vi "App - analyze RUS V6.vi"() -> ()   [LabVIEW 2021] (continued)
format"=enum."binary", "power(V)"=2.1, "Magn Field(T) "=0.0}, {"temperature"=67.561, "temperature str"="67.56100", "file path"=path "D:/Data/Ultrasound/LSCO/LSCO22__130814c/5_Cooling_2nd_try/September_2014/091714/67.56100K_500_2500_2.10000V_0.00000T_Sep17-2014__05-35-15_001_091714.bin", "last mod"=timestamp(3493791315 s since 1904-01-01), "file name str"="D:\\Data\\Ultrasound\\LSCO\\LSCO22__130814c\\5_Cooling_2nd_try\\September_2014\\091714\\67.56100K_500_2500_2.10000V_0.00000T_Sep17-2014__05-35-15_001_091714.bin", "mod time(min)"=58229855.25, "file format"=enum."binary", "power(V)"=2.1, "Magn Field(T) "=0.0}, {"temperature"=67.503, "temperature str"="67.50300", "file path"=path "D:/Data/Ultrasound/LSCO/LSCO22__130814c/5_Cooling_2nd_try/September_2014/091714/67.50300K_500_2500_2.10000V_0.00000T_Sep17-2014__05-36-34_001_091714.bin", "last mod"=timestamp(3493791394 s since 1904-01-01), "file name str"="D:\\Data\\Ultrasound\\LSCO\\LSCO22__130814c\\5_Cooling_2nd_try\\September_2014\\091714\\67.50300K_500_2500_2.10000V_0.00000T_Sep17-2014__05-36-34_001_091714.bin", "mod time(min)"=58229856.56666667, "file format"=enum."binary", "power(V)"=2.1, "Magn Field(T) "=0.0}, {"temperature"=67.441, "temperature str"="67.44100", "file path"=path "D:/Data/Ultrasound/LSCO/LSCO22__130814c/5_Cooling_2nd_try/September_2014/091714/67.44100K_500_2500_2.10000V_0.00000T_Sep17-2014__05-37-53_001_091714.bin", "last mod"=timestamp(3493791473 s since 1904-01-01), "file name str"="D:\\Data\\Ultrasound\\LSCO\\LSCO22__130814c\\5_Cooling_2nd_try\\September_2014\\091714\\67.44100K_500_2500_2.10000V_0.00000T_Sep17-2014__05-37-53_001_091714.bin", "mod time(min)"=58229857.88333333, "file format"=enum."binary", "power(V)"=2.1, "Magn Field(T) "=0.0}, {"temperature"=67.379, "temperature str"="67.37900", "file path"=path "D:/Data/Ultrasound/LSCO/LSCO22__130814c/5_Cooling_2nd_try/September_2014/091714/67.37900K_500_2500_2.10000V_0.00000T_Sep17-2014__05-39-13_001_091714.bin", "last mod"=timestamp(3493791553 s since 1904-01-01), "file name str"="D:\\Data\\Ultrasound\\LSCO\\LSCO22__130814c\\5_Cooling_2nd_try\\September_2014\\091714\\67.37900K_500_2500_2.10000V_0.00000T_Sep17-2014__05-39-13_001_091714.bin", "mod time(min)"=58229859.21666667, "file format"=enum."binary", "power(V)"=2.1, "Magn Field(T) "=0.0}, {"temperature"=67.322, "temperature str"="67.32200", "file path"=path "D:/Data/Ultrasound/LSCO/LSCO22__130814c/5_Cooling_2nd_try/September_2014/091714/67.32200K_500_2500_2.10000V_0.00000T_Sep17-2014__05-40-32_001_091714.bin", "last mod"=timestamp(3493791632 s since 1904-01-01), "file name str"="D:\\Data\\Ultrasound\\LSCO\\LSCO22__130814c\\5_Cooling_2nd_try\\September_2014\\091714\\67.32200K_500_2500_2.10000V_0.00000T_Sep17-2014__05-40-32_001_091714.bin", "mod time(min)"=58229860.53333333, "file format"=enum."binary", "power(V)"=2.1, "Magn Field(T) "=0.0}, {"temperature"=67.261, "temperature str"="67.26100", "file path"=path "D:/Data/Ultrasound/LSCO/LSCO22__130814c/5_Cooling_2nd_try/September_2014/091714/67.26100K_500_2500_2.10000V_0.00000T_Sep17-2014__05-41-51_001_091714.bin", "last mod"=timestamp(3493791711 s since 1904-01-01), "file name str"="D:\\Data\\Ultrasound\\LSCO\\LSCO22__130814c\\5_Cooling_2nd_try\\September_2014\\091714\\67.26100K_500_2500_2.10000V_0.00000T_Sep17-2014__05-41-51_001_091714.bin", "mod time(min)"=58229861.85, "file format"=enum."binary", "power(V)"=2.1, "Magn Field(T) "=0.0}, {"temperature"=67.202, "temperature str"="67.20200", "file path"=path "D:/Data/Ultrasound/LSCO/LSCO22__130814c/5_Cooling_2nd_try/September_2014/091714/67.20200K_500_2500_2.10000V_0.00000T_Sep17-2014__05-43-11_001_091714.bin", "last mod"=timestamp(3493791791 s since 1904-01-01), "file name str"="D:\\Data\\Ultrasound\\LSCO\\LSCO22__130814c\\5_Cooling_2nd_try\\September_2014\\091714\\67.20200K_500_2500_2.10000V_0.00000T_Sep17-2014__05-43-11_001_091714.bin", "mod time(min)"=58229863.18333333, "file format"=enum."binary", "power(V)"=2.1, "Magn Field(T) "=0.0}, {"temperature"=67.139, "temperature str"="67.13900", "file path"=path "D:/Data/Ultrasound/LSCO/LSCO22__130814c/5_Cooling_2nd_try/September_2014/091714/67.13900K_500_2500_2.10000V_0.00000T_Sep17-2014__05-44-30_001_091714.bin", "last mod"=timestamp(3493791870 s since 1904-01-01), "file name str"="D:\\Data\\Ultrasound\\LSCO\\LSCO22__130814c\\5_Cooling_2nd_try\\September_2014\\091714\\67.13900K_500_2500_2.10000V_0.00000T_Sep17-2014__05-44-30_001_091714.bin", "mod time(min)"=58229864.5, "file format"=enum."binary", "power(V)"=2.1, "Magn Field(T) "=0.0}, {"temperature"=67.079, "temperature str"="67.07900", "file path"=path "D:/Data/Ultrasound/LSCO/LSCO22__130814c/5_Cooling_2nd_try/September_2014/091714/67.07900K_500_2500_2.10000V_0.00000T_Sep17-2014__05-45-49_001_091714.bin", "last mod"=timestamp(3493791949 s since 1904-01-01), "file name str"="D:\\Data\\Ultrasound\\LSCO\\LSCO22__130814c\\5_Cooling_2nd_try\\September_2014\\091714\\67.07900K_500_2500_2.10000V_0.00000T_Sep17-2014__05-45-49_001_091714.bin", "mod time(min)"=58229865.81666667, "file format"=enum."binary", "power(V)"=2.1, "Magn Field(T) "=0.0}, {"temperature"=67.02, "temperature str"="67.02000", "file path"=path "D:/Data/Ultrasound/LSCO/LSCO22__130814c/5_Cooling_2nd_try/September_2014/091714/67.02000K_500_2500_2.10000V_0.00000T_Sep17-2014__05-47-09_001_091714.bin", "last mod"=timestamp(3493792029 s since 1904-01-01), "file name str"="D:\\Data\\Ultrasound\\LSCO\\LSCO22__130814c\\5_Cooling_2nd_try\\September_2014\\091714\\67.02000K_500_2500_2.10000V_0.00000T_Sep17-2014__05-47-09_001_091714.bin", "mod time(min)"=58229867.15, "file format"=enum."binary", "power(V)"=2.1, "Magn Field(T) "=0.0}, {"temperature"=66.959, "temperature str"="66.95900", "file path"=path "D:/Data/Ultrasound/LSCO/LSCO22__130814c/5_Cooling_2nd_try/September_2014/091714/66.95900K_500_2500_2.10000V_0.00000T_Sep17-2014__05-48-28_001_091714.bin", "last mod"=timestamp(3493792108 s since 1904-01-01), "file name str"="D:\\Data\\Ultrasound\\LSCO\\LSCO22__130814c\\5_Cooling_2nd_try\\September_2014\\091714\\66.95900K_500_2500_2.10000V_0.00000T_Sep17-2014__05-48-28_001_091714.bin", "mod time(min)"=58229868.46666667, "file format"=enum."binary", "power(V)"=2.1, "Magn Field(T) "=0.0}, {"temperature"=66.901, "temperature str"="66.90100", "file path"=path "D:/Data/Ultrasound/LSCO/LSCO22__130814c/5_Cooling_2nd_try/September_2014/091714/66.90100K_500_2500_2.10000V_0.00000T_Sep17-2014__05-49-47_001_091714.bin", "last mod"=timestamp(3493792187 s since 1904-01-01), "file name str"="D:\\Data\\Ultrasound\\LSCO\\LSCO22__130814c\\5_Cooling_2nd_try\\September_2014\\091714\\66.90100K_500_2500_2.10000V_0.00000T_Sep17-2014__05-49-47_001_091714.bin", "mod time(min)"=58229869.78333333, "file format"=enum."binary", "power(V)"=2.1, "Magn Field(T) "=0.0}, {"temperature"=66.841, "temperature str"="66.84100", "file path"=path "D:/Data/Ultrasound/LSCO/LSCO22__130814c/5_Cooling_2nd_try/September_2014/091714/66.84100K_500_2500_2.10000V_0.00000T_Sep17-2014__05-51-07_001_091714.bin", "last mod"=timestamp(3493792267 s since 1904-01-01), "file name str"="D:\\Data\\Ultrasound\\LSCO\\LSCO22__130814c\\5_Cooling_2nd_try\\September_2014\\091714\\66.84100K_500_2500_2.10000V_0.00000T_Sep17-2014__05-51-07_001_091714.bin", "mod time(min)"=58229871.11666667, "file format"=enum."binary", "power(V)"=2.1, "Magn Field(T) "=0.0}, {"temperature"=66.779, "temperature str"="66.77900", "file path"=path "D:/Data/Ultrasound/LSCO/LSCO22__130814c/5_Cooling_2nd_try/September_2014/091714/66.77900K_500_2500_2.10000V_0.00000T_Sep17-2014__05-52-26_001_091714.bin", "last mod"=timestamp(3493792346 s since 1904-01-01), "file name str"="D:\\Data\\Ultrasound\\LSCO\\LSCO22__130814c\\5_Cooling_2nd_try\\September_2014\\091714\\66.77900K_500_2500_2.10000V_0.00000T_Sep17-2014__05-52-26_001_091714.bin", "mod time(min)"=58229872.43333333, "file format"=enum."binary", "power(V)"=2.1, "Magn Field(T) "=0.0}, {"temperature"=66.721, "temperature str"="66.72100", "file path"=path "D:/Data/Ultrasound/LSCO/LSCO22__130814c/5_Cooling_2nd_try/September_2014/091714/66.72100K_500_2500_2.10000V_0.00000T_Sep17-2014__05-53-45_001_091714.bin", "last mod"=timestamp(3493792425 s since 1904-01-01), "file name str"="D:\\Data\\Ultrasound\\LSCO\\LSCO22__130814c\\5_Cooling_2nd_try\\September_2014\\091714\\66.72100K_500_2500_2.10000V_0.00000T_Sep17-2014__05-53-45_001_091714.bin", "mod time(min)"=58229873.75, "file format"=enum."binary", "power(V)"=2.1, "Magn Field(T) "=0.0}, {"temperature"=66.66, "temperature str"="66.66000", "file path"=path "D:/Data/Ultrasound/LSCO/LSCO22__130814c/5_Cooling_2nd_try/September_2014/091714/66.66000K_500_2500_2.10000V_0.00000T_Sep17-2014__05-55-05_001_091714.bin", "last mod"=timestamp(3493792505 s since 1904-01-01), "file name str"="D:\\Data\\Ultrasound\\LSCO\\LSCO22__130814c\\5_Cooling_2nd_try\\September_2014\\091714\\66.66000K_500_2500_2.10000V_0.00000T_Sep17-2014__05-55-05_001_091714.bin", "mod time(min)"=58229875.083333336, "file format"=enum."binary", "power(V)"=2.1, "Magn Field(T) "=0.0}, {"temperature"=66.601, "temperature str"="66.60100", "file path"=path "D:/Data/Ultrasound/LSCO/LSCO22__130814c/5_Cooling_2nd_try/September_2014/091714/66.60100K_500_2500_2.10000V_0.00000T_Sep17-2014__05-56-24_001_091714.bin", "last mod"=timestamp(3493792584 s since 1904-01-01), "file name str"="D:\\Data\\Ultrasound\\LSCO\\LSCO22__130814c\\5_Cooling_2nd_try\\September_2014\\091714\\66.60100K_500_2500_2.10000V_0.00000T_Sep17-2014__05-56-24_001_091714.bin", "mod time(min)"=58229876.4, "file format"=enum."binary", "power(V)"=2.1, "Magn Field(T) "=0.0}, {"temperature"=66.541, "temperature str"="66.54100", "file path"=path "D:/Data/Ultrasound/LSCO/LSCO22__130814c/5_Cooling_2nd_try/September_2014/091714/66.54100K_500_2500_2.10000V_0.00000T_Sep17-2014__05-57-44_001_091714.bin", "last mod"=timestamp(3493792664 s since 1904-01-01), "file name str"="D:\\Data\\Ultrasound\\LSCO\\LSCO22__130814c\\5_Cooling_2nd_try\\September_2014\\091714\\66.54100K_500_2500_2.10000V_0.00000T_Sep17-2014__05-57-44_001_091714.bin", "mod time(min)"=58229877.733333334, "file format"=enum."binary", "power(V)"=2.1, "Magn Field(T) "=0.0}, {"temperature"=66.48, "temperature str"="66.48000", "file path"=path "D:/Data/Ultrasound/LSCO/LSCO22__130814c/5_Cooling_2nd_try/September_2014/091714/66.48000K_500_2500_2.10000V_0.00000T_Sep17-2014__05-59-03_001_091714.bin", "last mod"=timestamp(3493792743 s since 1904-01-01), "file name str"="D:\\Data\\Ultrasound\\LSCO\\LSCO22__130814c\\5_Cooling_2nd_try\\September_2014\\091714\\66.48000K_500_2500_2.10000V_0.00000T_Sep17-2014__05-59-03_001_091714.bin", "mod time(min)"=58229879.05, "file format"=enum."binary", "power(V)"=2.1, "Magn Field(T) "=0.0}, {"temperature"=66.422, "temperature str"="66.42200", "file path"=path "D:/Data/Ultrasound/LSCO/LSCO22__130814c/5_Cooling_2nd_try/September_2014/091714/66.42200K_500_2500_2.10000V_0.00000T_Sep17-2014__06-00-22_001_091714.bin", "last mod"=timestamp(3493792822 s since 1904-01-01), "file name str"="D:\\Data\\Ultrasound\\LSCO\\LSCO22__130814c\\5_Cooling_2nd_try\\September_2014\\091714\\66.42200K_500_2500_2.10000V_0.00000T_Sep17-2014__06-00-22_001_091714.bin", "mod time(min)"=58229880.36666667, "file format"=enum."binary", "power(V)"=2.1, "Magn Field(T) "=0.0}, {"temperature"=66.363, "temperature str"="66.36300", "file path"=path "D:/Data/Ultrasound/LSCO/LSCO22__130814c/5_Cooling_2nd_try/September_2014/091714/66.36300K_500_2500_2.10000V_0.00000T_Sep17-2014__06-01-42_001_091714.bin", "last mod"=timestamp(3493792902 s since 1904-01-01), "file name str"="D:\\Data\\Ultrasound\\LSCO\\LSCO22__130814c\\5_Cooling_2nd_try\\September_2014\\091714\\66.36300K_500_2500_2.10000V_0.00000T_Sep17-2014__06-01-42_001_091714.bin", "mod time(min)"=58229881.7, "file format"=enum."binary", "power(V)"=2.1, "Magn Field(T) "=0.0}, {"temperature"=66.302, "temperature str"="66.30200", "file path"=path "D:/Data/Ultrasound/LSCO/LSCO22__130814c/5_Cooling_2nd_try/September_2014/091714/66.30200K_500_2500_2.10000V_0.00000T_Sep17-2014__06-03-01_001_091714.bin", "last mod"=timestamp(3493792981 s since 1904-01-01), "file name str"="D:\\Data\\Ultrasound\\LSCO\\LSCO22__130814c\\5_Cooling_2nd_try\\September_2014\\091714\\66.30200K_500_2500_2.10000V_0.00000T_Sep17-2014__06-03-01_001_091714.bin", "mod time(min)"=58229883.016666666, "file format"=enum."binary", "power(V)"=2.1, "Magn Field(T) "=0.0}, {"temperature"=66.244, "temperature str"="66.24400", "file path"=path "D:/Data/Ultrasound/LSCO/LSCO22__130814c/5_Cooling_2nd_try/September_2014/091714/66.24400K_500_2500_2.10000V_0.00000T_Sep17-2014__06-04-20_001_091714.bin", "last mod"=timestamp(3493793060 s since 1904-01-01), "file name str"="D:\\Data\\Ultrasound\\LSCO\\LSCO22__130814c\\5_Cooling_2nd_try\\September_2014\\091714\\66.24400K_500_2500_2.10000V_0.00000T_Sep17-2014__06-04-20_001_091714.bin", "mod time(min)"=58229884.333333336, "file format"=enum."binary", "power(V)"=2.1, "Magn Field(T) "=0.0}, {"temperature"=66.182, "temperature str"="66.18200", "file path"=path "D:/Data/Ultrasound/LSCO/LSCO22__130814c/5_Cooling_2nd_try/September_2014/091714/66.18200K_500_2500_2.10000V_0.00000T_Sep17-2014__06-05-40_001_091714.bin", "last mod"=timestamp(3493793140 s since 1904-01-01), "file name str"="D:\\Data\\Ultrasound\\LSCO\\LSCO22__130814c\\5_Cooling_2nd_try\\September_2014\\091714\\66.18200K_500_2500_2.10000V_0.00000T_Sep17-2014__06-05-40_001_091714.bin", "mod time(min)"=58229885.666666664, "file format"=enum."binary", "power(V)"=2.1, "Magn Field(T) "=0.0}, {"temperature"=66.124, "temperature str"="66.12400", "file path"=path "D:/Data/Ultrasound/LSCO/LSCO22__130814c/5_Cooling_2nd_try/September_2014/091714/66.12400K_500_2500_2.10000V_0.00000T_Sep17-2014__06-06-59_001_091714.bin", "last mod"=timestamp(3493793219 s since 1904-01-01), "file name str"="D:\\Data\\Ultrasound\\LSCO\\LSCO22__130814c\\5_Cooling_2nd_try\\September_2014\\091714\\66.12400K_500_2500_2.10000V_0.00000T_Sep17-2014__06-06-59_001_091714.bin", "mod time(min)"=58229886.983333334, "file format"=enum."binary", "power(V)"=2.1, "Magn Field(T) "=0.0}, {"temperature"=66.063, "temperature str"="66.06300", "file path"=path "D:/Data/Ultrasound/LSCO/LSCO22__130814c/5_Cooling_2nd_try/September_2014/091714/66.06300K_500_2500_2.10000V_0.00000T_Sep17-2014__06-08-19_001_091714.bin", "last mod"=timestamp(3493793299 s since 1904-01-01), "file name str"="D:\\Data\\Ultrasound\\LSCO\\LSCO22__130814c\\5_Cooling_2nd_try\\September_2014\\091714\\66.06300K_500_2500_2.10000V_0.00000T_Sep17-2014__06-08-19_001_091714.bin", "mod time(min)"=58229888.31666667, "file format"=enum."binary", "power(V)"=2.1, "Magn Field(T) "=0.0}, {"temperature"=66.006, "temperature str"="66.00600", "file path"=path "D:/Data/Ultrasound/LSCO/LSCO22__130814c/5_Cooling_2nd_try/September_2014/091714/66.00600K_500_2500_2.10000V_0.00000T_Sep17-2014__06-09-38_001_091714.bin", "last mod"=timestamp(3493793378 s since 1904-01-01), "file name str"="D:\\Data\\Ultrasound\\LSCO\\LSCO22__130814c\\5_Cooling_2nd_try\\September_2014\\091714\\66.00600K_500_2500_2.10000V_0.00000T_Sep17-2014__06-09-38_001_091714.bin", "mod time(min)"=58229889.63333333, "file format"=enum."binary", "power(V)"=2.1, "Magn Field(T) "=0.0}, {"temperature"=65.947, "temperature str"="65.94700", "file path"=path "D:/Data/Ultrasound/LSCO/LSCO22__130814c/5_Cooling_2nd_try/September_2014/091714/65.94700K_500_2500_2.10000V_0.00000T_Sep17-2014__06-10-57_001_091714.bin", "last mod"=timestamp(3493793457 s since 1904-01-01), "file name str"="D:\\Data\\Ultrasound\\LSCO\\LSCO22__130814c\\5_Cooling_2nd_try\\September_2014\\091714\\65.94700K_500_2500_2.10000V_0.00000T_Sep17-2014__06-10-57_001_091714.bin", "mod time(min)"=58229890.95, "file format"=enum."binary", "power(V)"=2.1, "Magn Field(T) "=0.0}, {"temperature"=65.884, "temperature str"="65.88400", "file path"=path "D:/Data/Ultrasound/LSCO/LSCO22__130814c/5_Cooling_2nd_try/September_2014/091714/65.88400K_500_2500_2.10000V_0.00000T_Sep17-2014__06-12-17_001_091714.bin", "last mod"=timestamp(3493793537 s since 1904-01-01), "file name str"="D:\\Data\\Ultrasound\\LSCO\\LSCO22__130814c\\5_Cooling_2nd_try\\September_2014\\091714\\65.88400K_500_2500_2.10000V_0.00000T_Sep17-2014__06-12-17_001_091714.bin", "mod time(min)"=58229892.28333333, "file format"=enum."binary", "power(V)"=2.1, "Magn Field(T) "=0.0}, {"temperature"=65.828, "temperature str"="65.82800", "file path"=path "D:/Data/Ultrasound/LSCO/LSCO22__130814c/5_Cooling_2nd_try/September_2014/091714/65.82800K_500_2500_2.10000V_0.00000T_Sep17-2014__06-13-36_001_091714.bin", "last mod"=timestamp(3493793616 s since 1904-01-01), "file name str"="D:\\Data\\Ultrasound\\LSCO\\LSCO22__130814c\\5_Cooling_2nd_try\\September_2014\\091714\\65.82800K_500_2500_2.10000V_0.00000T_Sep17-2014__06-13-36_001_091714.bin", "mod time(min)"=58229893.6, "file format"=enum."binary", "power(V)"=2.1, "Magn Field(T) "=0.0}, {"temperature"=65.767, "temperature str"="65.76700", "file path"=path "D:/Data/Ultrasound/LSCO/LSCO22__130814c/5_Cooling_2nd_try/September_2014/091714/65.76700K_500_2500_2.10000V_0.00000T_Sep17-2014__06-14-56_001_091714.bin", "last mod"=timestamp(3493793696 s since 1904-01-01), "file name str"="D:\\Data\\Ultrasound\\LSCO\\LSCO22__130814c\\5_Cooling_2nd_try\\September_2014\\091714\\65.76700K_500_2500_2.10000V_0.00000T_Sep17-2014__06-14-56_001_091714.bin", "mod time(min)"=58229894.93333333, "file format"=enum."binary", "power(V)"=2.1, "Magn Field(T) "=0.0}, {"temperature"=65.71, "temperature str"="65.71000", "file path"=path "D:/Data/Ultrasound/LSCO/LSCO22__130814c/5_Cooling_2nd_try/September_2014/091714/65.71000K_500_2500_2.10000V_0.00000T_Sep17-2014__06-16-15_001_091714.bin", "last mod"=timestamp(3493793775 s since 1904-01-01), "file name str"="D:\\Data\\Ultrasound\\LSCO\\LSCO22__130814c\\5_Cooling_2nd_try\\September_2014\\091714\\65.71000K_500_2500_2.10000V_0.00000T_Sep17-2014__06-16-15_001_091714.bin", "mod time(min)"=58229896.25, "file format"=enum."binary", "power(V)"=2.1, "Magn Field(T) "=0.0}, {"temperature"=65.648, "temperature str"="65.64800", "file path"=path "D:/Data/Ultrasound/LSCO/LSCO22__130814c/5_Cooling_2nd_try/September_2014/091714/65.64800K_500_2500_2.10000V_0.00000T_Sep17-2014__06-17-34_001_091714.bin", "last mod"=timestamp(3493793854 s since 1904-01-01), "file name str"="D:\\Data\\Ultrasound\\LSCO\\LSCO22__130814c\\5_Cooling_2nd_try\\September_2014\\091714\\65.64800K_500_2500_2.10000V_0.00000T_Sep17-2014__06-17-34_001_091714.bin", "mod time(min)"=58229897.56666667, "file format"=enum."binary", "power(V)"=2.1, "Magn Field(T) "=0.0}, {"temperature"=65.588, "temperature str"="65.58800", "file path"=path "D:/Data/Ultrasound/LSCO/LSCO22__130814c/5_Cooling_2nd_try/September_2014/091714/65.58800K_500_2500_2.10000V_0.00000T_Sep17-2014__06-18-54_001_091714.bin", "last mod"=timestamp(3493793934 s since 1904-01-01), "file name str"="D:\\Data\\Ultrasound\\LSCO\\LSCO22__130814c\\5_Cooling_2nd_try\\September_2014\\091714\\65.58800K_500_2500_2.10000V_0.00000T_Sep17-2014__06-18-54_001_091714.bin", "mod time(min)"=58229898.9, "file format"=enum."binary", "power(V)"=2.1, "Magn Field(T) "=0.0}, {"temperature"=65.531, "temperature str"="65.53100", "file path"=path "D:/Data/Ultrasound/LSCO/LSCO22__130814c/5_Cooling_2nd_try/September_2014/091714/65.53100K_500_2500_2.10000V_0.00000T_Sep17-2014__06-20-13_001_091714.bin", "last mod"=timestamp(3493794013 s since 1904-01-01), "file name str"="D:\\Data\\Ultrasound\\LSCO\\LSCO22__130814c\\5_Cooling_2nd_try\\September_2014\\091714\\65.53100K_500_2500_2.10000V_0.00000T_Sep17-2014__06-20-13_001_091714.bin", "mod time(min)"=58229900.21666667, "file format"=enum."binary", "power(V)"=2.1, "Magn Field(T) "=0.0}, {"temperature"=65.472, "temperature str"="65.47200", "file path"=path "D:/Data/Ultrasound/LSCO/LSCO22__130814c/5_Cooling_2nd_try/September_2014/091714/65.47200K_500_2500_2.10000V_0.00000T_Sep17-2014__06-21-32_001_091714.bin", "last mod"=timestamp(3493794092 s since 1904-01-01), "file name str"="D:\\Data\\Ultrasound\\LSCO\\LSCO22__130814c\\5_Cooling_2nd_try\\September_2014\\091714\\65.47200K_500_2500_2.10000V_0.00000T_Sep17-2014__06-21-32_001_091714.bin", "mod time(min)"=58229901.53333333, "file format"=enum."binary", "power(V)"=2.1, "Magn Field(T) "=0.0}, {"temperature"=65.412, "temperature str"="65.41200", "file path"=path "D:/Data/Ultrasound/LSCO/LSCO22__130814c/5_Cooling_2nd_try/September_2014/091714/65.41200K_500_2500_2.10000V_0.00000T_Sep17-2014__06-22-52_001_091714.bin", "last mod"=timestamp(3493794172 s since 1904-01-01), "file name str"="D:\\Data\\Ultrasound\\LSCO\\LSCO22__130814c\\5_Cooling_2nd_try\\September_2014\\091714\\65.41200K_500_2500_2.10000V_0.00000T_Sep17-2014__06-22-52_001_091714.bin", "mod time(min)"=58229902.86666667, "file format"=enum."binary", "power(V)"=2.1, "Magn Field(T) "=0.0}, {"temperature"=65.354, "temperature str"="65.35400", "file path"=path "D:/Data/Ultrasound/LSCO/LSCO22__130814c/5_Cooling_2nd_try/September_2014/091714/65.35400K_500_2500_2.10000V_0.00000T_Sep17-2014__06-24-11_001_091714.bin", "last mod"=timestamp(3493794251 s since 1904-01-01), "file name str"="D:\\Data\\Ultrasound\\LSCO\\LSCO22__130814c\\5_Cooling_2nd_try\\September_2014\\091714\\65.35400K_500_2500_2.10000V_0.00000T_Sep17-2014__06-24-11_001_091714.bin", "mod time(min)"=58229904.18333333, "file format"=enum."binary", "power(V)"=2.1, "Magn Field(T) "=0.0}, {"temperature"=65.294, "temperature str"="65.29400", "file path"=path "D:/Data/Ultrasound/LSCO/LSCO22__130814c/5_Cooling_2nd_try/September_2014/091714/65.29400K_500_2500_2.10000V_0.00000T_Sep17-2014__06-25-31_001_091714.bin", "last mod"=timestamp(3493794331 s since 1904-01-01), "file name str"="D:\\Data\\Ultrasound\\LSCO\\LSCO22__130814c\\5_Cooling_2nd_try\\September_2014\\091714\\65.29400K_500_2500_2.10000V_0.00000T_Sep17-2014__06-25-31_001_091714.bin", "mod time(min)"=58229905.516666666, "file format"=enum."binary", "power(V)"=2.1, "Magn Field(T) "=0.0}, {"temperature"=65.236, "temperature str"="65.23600", "file path"=path "D:/Data/Ultrasound/LSCO/LSCO22__130814c/5_Cooling_2nd_try/September_2014/091714/65.23600K_500_2500_2.10000V_0.00000T_Sep17-2014__06-26-50_001_091714.bin", "last mod"=timestamp(3493794410 s since 1904-01-01), "file name str"="D:\\Data\\Ultrasound\\LSCO\\LSCO22__130814c\\5_Cooling_2nd_try\\September_2014\\091714\\65.23600K_500_2500_2.10000V_0.00000T_Sep17-2014__06-26-50_001_091714.bin", "mod time(min)"=58229906.833333336, "file format"=enum."binary", "power(V)"=2.1, "Magn Field(T) "=0.0}, {"temperature"=65.176, "temperature str"="65.17600", "file path"=path "D:/Data/Ultrasound/LSCO/LSCO22__130814c/5_Cooling_2nd_try/September_2014/091714/65.17600K_500_2500_2.10000V_0.00000T_Sep17-2014__06-28-09_001_091714.bin", "last mod"=timestamp(3493794489 s since 1904-01-01), "file name str"="D:\\Data\\Ultrasound\\LSCO\\LSCO22__130814c\\5_Cooling_2nd_try\\September_2014\\091714\\65.17600K_500_2500_2.10000V_0.00000T_Sep17-2014__06-28-09_001_091714.bin", "mod time(min)"=58229908.15, "file format"=enum."binary", "power(V)"=2.1, "Magn Field(T) "=0.0}, {"temperature"=65.115, "temperature str"="65.11500", "file path"=path "D:/Data/Ultrasound/LSCO/LSCO22__130814c/5_Cooling_2nd_try/September_2014/091714/65.11500K_500_2500_2.10000V_0.00000T_Sep17-2014__06-29-29_001_091714.bin", "last mod"=timestamp(3493794569 s since 1904-01-01), "file name str"="D:\\Data\\Ultrasound\\LSCO\\LSCO22__130814c\\5_Cooling_2nd_try\\September_2014\\091714\\65.11500K_500_2500_2.10000V_0.00000T_Sep17-2014__06-29-29_001_091714.bin", "mod time(min)"=58229909.483333334, "file format"=enum."binary", "power(V)"=2.1, "Magn Field(T) "=0.0}, {"temperature"=65.059, "temperature str"="65.05900", "file path"=path "D:/Data/Ultrasound/LSCO/LSCO22__130814c/5_Cooling_2nd_try/September_2014/091714/65.05900K_500_2500_2.10000V_0.00000T_Sep17-2014__06-30-48_001_091714.bin", "last mod"=timestamp(3493794648 s since 1904-01-01), "file name str"="D:\\Data\\Ultrasound\\LSCO\\LSCO22__130814c\\5_Cooling_2nd_try\\September_2014\\091714\\65.05900K_500_2500_2.10000V_0.00000T_Sep17-2014__06-30-48_001_091714.bin", "mod time(min)"=58229910.8, "file format"=enum."binary", "power(V)"=2.1, "Magn Field(T) "=0.0}, {"temperature"=64.997, "temperature str"="64.99700", "file path"=path "D:/Data/Ultrasound/LSCO/LSCO22__130814c/5_Cooling_2nd_try/September_2014/091714/64.99700K_500_2500_2.10000V_0.00000T_Sep17-2014__06-32-08_001_091714.bin", "last mod"=timestamp(3493794728 s since 1904-01-01), "file name str"="D:\\Data\\Ultrasound\\LSCO\\LSCO22__130814c\\5_Cooling_2nd_try\\September_2014\\091714\\64.99700K_500_2500_2.10000V_0.00000T_Sep17-2014__06-32-08_001_091714.bin", "mod time(min)"=58229912.13333333, "file format"=enum."binary", "power(V)"=2.1, "Magn Field(T) "=0.0}, {"temperature"=64.94, "temperature str"="64.94000", "file path"=path "D:/Data/Ultrasound/LSCO/LSCO22__130814c/5_Cooling_2nd_try/September_2014/091714/64.94000K_500_2500_2.10000V_0.00000T_Sep17-2014__06-33-27_001_091714.bin", "last mod"=timestamp(3493794807 s since 1904-01-01), "file name str"="D:\\Data\\Ultrasound\\LSCO\\LSCO22__130814c\\5_Cooling_2nd_try\\September_2014\\091714\\64.94000K_500_2500_2.10000V_0.00000T_Sep17-2014__06-33-27_001_091714.bin", "mod time(min)"=58229913.45, "file format"=enum."binary", "power(V)"=2.1, "Magn Field(T) "=0.0}, {"temperature"=64.883, "temperature str"="64.88300", "file path"=path "D:/Data/Ultrasound/LSCO/LSCO22__130814c/5_Cooling_2nd_try/September_2014/091714/64.88300K_500_2500_2.10000V_0.00000T_Sep17-2014__06-34-46_001_091714.bin", "last mod"=timestamp(3493794886 s since 1904-01-01), "file name str"="D:\\Data\\Ultrasound\\LSCO\\LSCO22__130814c\\5_Cooling_2nd_try\\September_2014\\091714\\64.88300K_500_2500_2.10000V_0.00000T_Sep17-2014__06-34-46_001_091714.bin", "mod time(min)"=58229914.766666666, "file format"=enum."binary", "power(V)"=2.1, "Magn Field(T) "=0.0}, {"temperature"=64.821, "temperature str"="64.82100", "file path"=path "D:/Data/Ultrasound/LSCO/LSCO22__130814c/5_Cooling_2nd_try/September_2014/091714/64.82100K_500_2500_2.10000V_0.00000T_Sep17-2014__06-36-06_001_091714.bin", "last mod"=timestamp(3493794966 s since 1904-01-01), "file name str"="D:\\Data\\Ultrasound\\LSCO\\LSCO22__130814c\\5_Cooling_2nd_try\\September_2014\\091714\\64.82100K_500_2500_2.10000V_0.00000T_Sep17-2014__06-36-06_001_091714.bin", "mod time(min)"=58229916.1, "file format"=enum."binary", "power(V)"=2.1, "Magn Field(T) "=0.0}, {"temperature"=64.764, "temperature str"="64.76400", "file path"=path "D:/Data/Ultrasound/LSCO/LSCO22__130814c/5_Cooling_2nd_try/September_2014/091714/64.76400K_500_2500_2.10000V_0.00000T_Sep17-2014__06-37-25_001_091714.bin", "last mod"=timestamp(3493795045 s since 1904-01-01), "file name str"="D:\\Data\\Ultrasound\\LSCO\\LSCO22__130814c\\5_Cooling_2nd_try\\September_2014\\091714\\64.76400K_500_2500_2.10000V_0.00000T_Sep17-2014__06-37-25_001_091714.bin", "mod time(min)"=58229917.416666664, "file format"=enum."binary", "power(V)"=2.1, "Magn Field(T) "=0.0}, {"temperature"=64.703, "temperature str"="64.70300", "file path"=path "D:/Data/Ultrasound/LSCO/LSCO22__130814c/5_Cooling_2nd_try/September_2014/091714/64.70300K_500_2500_2.10000V_0.00000T_Sep17-2014__06-38-44_001_091714.bin", "last mod"=timestamp(3493795124 s since 1904-01-01), "file name str"="D:\\Data\\Ultrasound\\LSCO\\LSCO22__130814c\\5_Cooling_2nd_try\\September_2014\\091714\\64.70300K_500_2500_2.10000V_0.00000T_Sep17-2014__06-38-44_001_091714.bin", "mod time(min)"=58229918.733333334, "file format"=enum."binary", "power(V)"=2.1, "Magn Field(T) "=0.0}, {"temperature"=64.649, "temperature str"="64.64900", "file path"=path "D:/Data/Ultrasound/LSCO/LSCO22__130814c/5_Cooling_2nd_try/September_2014/091714/64.64900K_500_2500_2.10000V_0.00000T_Sep17-2014__06-40-04_001_091714.bin", "last mod"=timestamp(3493795204 s since 1904-01-01), "file name str"="D:\\Data\\Ultrasound\\LSCO\\LSCO22__130814c\\5_Cooling_2nd_try\\September_2014\\091714\\64.64900K_500_2500_2.10000V_0.00000T_Sep17-2014__06-40-04_001_091714.bin", "mod time(min)"=58229920.06666667, "file format"=enum."binary", "power(V)"=2.1, "Magn Field(T) "=0.0}, {"temperature"=64.588, "temperature str"="64.58800", "file path"=path "D:/Data/Ultrasound/LSCO/LSCO22__130814c/5_Cooling_2nd_try/September_2014/091714/64.58800K_500_2500_2.10000V_0.00000T_Sep17-2014__06-41-23_001_091714.bin", "last mod"=timestamp(3493795283 s since 1904-01-01), "file name str"="D:\\Data\\Ultrasound\\LSCO\\LSCO22__130814c\\5_Cooling_2nd_try\\September_2014\\091714\\64.58800K_500_2500_2.10000V_0.00000T_Sep17-2014__06-41-23_001_091714.bin", "mod time(min)"=58229921.38333333, "file format"=enum."binary", "power(V)"=2.1, "Magn Field(T) "=0.0}, {"temperature"=64.527, "temperature str"="64.52700", "file path"=path "D:/Data/Ultrasound/LSCO/LSCO22__130814c/5_Cooling_2nd_try/September_2014/091714/64.52700K_500_2500_2.10000V_0.00000T_Sep17-2014__06-42-43_001_091714.bin", "last mod"=timestamp(3493795363 s since 1904-01-01), "file name str"="D:\\Data\\Ultrasound\\LSCO\\LSCO22__130814c\\5_Cooling_2nd_try\\September_2014\\091714\\64.52700K_500_2500_2.10000V_0.00000T_Sep17-2014__06-42-43_001_091714.bin", "mod time(min)"=58229922.71666667, "file format"=enum."binary", "power(V)"=2.1, "Magn Field(T) "=0.0}, {"temperature"=64.473, "temperature str"="64.47300", "file path"=path "D:/Data/Ultrasound/LSCO/LSCO22__130814c/5_Cooling_2nd_try/September_2014/091714/64.47300K_500_2500_2.10000V_0.00000T_Sep17-2014__06-44-02_001_091714.bin", "last mod"=timestamp(3493795442 s since 1904-01-01), "file name str"="D:\\Data\\Ultrasound\\LSCO\\LSCO22__130814c\\5_Cooling_2nd_try\\September_2014\\091714\\64.47300K_500_2500_2.10000V_0.00000T_Sep17-2014__06-44-02_001_091714.bin", "mod time(min)"=58229924.03333333, "file format"=enum."binary", "power(V)"=2.1, "Magn Field(T) "=0.0}, {"temperature"=64.413, "temperature str"="64.41300", "file path"=path "D:/Data/Ultrasound/LSCO/LSCO22__130814c/5_Cooling_2nd_try/September_2014/091714/64.41300K_500_2500_2.10000V_0.00000T_Sep17-2014__06-45-21_001_091714.bin", "last mod"=timestamp(3493795521 s since 1904-01-01), "file name str"="D:\\Data\\Ultrasound\\LSCO\\LSCO22__130814c\\5_Cooling_2nd_try\\September_2014\\091714\\64.41300K_500_2500_2.10000V_0.00000T_Sep17-2014__06-45-21_001_091714.bin", "mod time(min)"=58229925.35, "file format"=enum."binary", "power(V)"=2.1, "Magn Field(T) "=0.0}, {"temperature"=64.354, "temperature str"="64.35400", "file path"=path "D:/Data/Ultrasound/LSCO/LSCO22__130814c/5_Cooling_2nd_try/September_2014/091714/64.35400K_500_2500_2.10000V_0.00000T_Sep17-2014__06-46-41_001_091714.bin", "last mod"=timestamp(3493795601 s since 1904-01-01), "file name str"="D:\\Data\\Ultrasound\\LSCO\\LSCO22__130814c\\5_Cooling_2nd_try\\September_2014\\091714\\64.35400K_500_2500_2.10000V_0.00000T_Sep17-2014__06-46-41_001_091714.bin", "mod time(min)"=58229926.68333333, "file format"=enum."binary", "power(V)"=2.1, "Magn Field(T) "=0.0}, {"temperature"=64.292, "temperature str"="64.29200", "file path"=path "D:/Data/Ultrasound/LSCO/LSCO22__130814c/5_Cooling_2nd_try/September_2014/091714/64.29200K_500_2500_2.10000V_0.00000T_Sep17-2014__06-48-00_001_091714.bin", "last mod"=timestamp(3493795680 s since 1904-01-01), "file name str"="D:\\Data\\Ultrasound\\LSCO\\LSCO22__130814c\\5_Cooling_2nd_try\\September_2014\\091714\\64.29200K_500_2500_2.10000V_0.00000T_Sep17-2014__06-48-00_001_091714.bin", "mod time(min)"=58229928.0, "file format"=enum."binary", "power(V)"=2.1, "Magn Field(T) "=0.0}, {"temperature"=64.234, "temperature str"="64.23400", "file path"=path "D:/Data/Ultrasound/LSCO/LSCO22__130814c/5_Cooling_2nd_try/September_2014/091714/64.23400K_500_2500_2.10000V_0.00000T_Sep17-2014__06-49-20_001_091714.bin", "last mod"=timestamp(3493795760 s since 1904-01-01), "file name str"="D:\\Data\\Ultrasound\\LSCO\\LSCO22__130814c\\5_Cooling_2nd_try\\September_2014\\091714\\64.23400K_500_2500_2.10000V_0.00000T_Sep17-2014__06-49-20_001_091714.bin", "mod time(min)"=58229929.333333336, "file format"=enum."binary", "power(V)"=2.1, "Magn Field(T) "=0.0}, {"temperature"=64.177, "temperature str"="64.17700", "file path"=path "D:/Data/Ultrasound/LSCO/LSCO22__130814c/5_Cooling_2nd_try/September_2014/091714/64.17700K_500_2500_2.10000V_0.00000T_Sep17-2014__06-50-39_001_091714.bin", "last mod"=timestamp(3493795839 s since 1904-01-01), "file name str"="D:\\Data\\Ultrasound\\LSCO\\LSCO22__130814c\\5_Cooling_2nd_try\\September_2014\\091714\\64.17700K_500_2500_2.10000V_0.00000T_Sep17-2014__06-50-39_001_091714.bin", "mod time(min)"=58229930.65, "file format"=enum."binary", "power(V)"=2.1, "Magn Field(T) "=0.0}, {"temperature"=64.117, "temperature str"="64.11700", "file path"=path "D:/Data/Ultrasound/LSCO/LSCO22__130814c/5_Cooling_2nd_try/September_2014/091714/64.11700K_500_2500_2.10000V_0.00000T_Sep17-2014__06-51-58_001_091714.bin", "last mod"=timestamp(3493795918 s since 1904-01-01), "file name str"="D:\\Data\\Ultrasound\\LSCO\\LSCO22__130814c\\5_Cooling_2nd_try\\September_2014\\091714\\64.11700K_500_2500_2.10000V_0.00000T_Sep17-2014__06-51-58_001_091714.bin", "mod time(min)"=58229931.96666667, "file format"=enum."binary", "power(V)"=2.1, "Magn Field(T) "=0.0}, {"temperature"=64.06, "temperature str"="64.06000", "file path"=path "D:/Data/Ultrasound/LSCO/LSCO22__130814c/5_Cooling_2nd_try/September_2014/091714/64.06000K_500_2500_2.10000V_0.00000T_Sep17-2014__06-53-18_001_091714.bin", "last mod"=timestamp(3493795998 s since 1904-01-01), "file name str"="D:\\Data\\Ultrasound\\LSCO\\LSCO22__130814c\\5_Cooling_2nd_try\\September_2014\\091714\\64.06000K_500_2500_2.10000V_0.00000T_Sep17-2014__06-53-18_001_091714.bin", "mod time(min)"=58229933.3, "file format"=enum."binary", "power(V)"=2.1, "Magn Field(T) "=0.0}, {"temperature"=64.001, "temperature str"="64.00100", "file path"=path "D:/Data/Ultrasound/LSCO/LSCO22__130814c/5_Cooling_2nd_try/September_2014/091714/64.00100K_500_2500_2.10000V_0.00000T_Sep17-2014__06-54-37_001_091714.bin", "last mod"=timestamp(3493796077 s since 1904-01-01), "file name str"="D:\\Data\\Ultrasound\\LSCO\\LSCO22__130814c\\5_Cooling_2nd_try\\September_2014\\091714\\64.00100K_500_2500_2.10000V_0.00000T_Sep17-2014__06-54-37_001_091714.bin", "mod time(min)"=58229934.61666667, "file format"=enum."binary", "power(V)"=2.1, "Magn Field(T) "=0.0}, {"temperature"=63.941, "temperature str"="63.94100", "file path"=path "D:/Data/Ultrasound/LSCO/LSCO22__130814c/5_Cooling_2nd_try/September_2014/091714/63.94100K_500_2500_2.10000V_0.00000T_Sep17-2014__06-55-56_001_091714.bin", "last mod"=timestamp(3493796156 s since 1904-01-01), "file name str"="D:\\Data\\Ultrasound\\LSCO\\LSCO22__130814c\\5_Cooling_2nd_try\\September_2014\\091714\\63.94100K_500_2500_2.10000V_0.00000T_Sep17-2014__06-55-56_001_091714.bin", "mod time(min)"=58229935.93333333, "file format"=enum."binary", "power(V)"=2.1, "Magn Field(T) "=0.0}, {"temperature"=63.884, "temperature str"="63.88400", "file path"=path "D:/Data/Ultrasound/LSCO/LSCO22__130814c/5_Cooling_2nd_try/September_2014/091714/63.88400K_500_2500_2.10000V_0.00000T_Sep17-2014__06-57-16_001_091714.bin", "last mod"=timestamp(3493796236 s since 1904-01-01), "file name str"="D:\\Data\\Ultrasound\\LSCO\\LSCO22__130814c\\5_Cooling_2nd_try\\September_2014\\091714\\63.88400K_500_2500_2.10000V_0.00000T_Sep17-2014__06-57-16_001_091714.bin", "mod time(min)"=58229937.266666666, "file format"=enum."binary", "power(V)"=2.1, "Magn Field(T) "=0.0}, {"temperature"=63.822, "temperature str"="63.82200", "file path"=path "D:/Data/Ultrasound/LSCO/LSCO22__130814c/5_Cooling_2nd_try/September_2014/091714/63.82200K_500_2500_2.10000V_0.00000T_Sep17-2014__06-58-35_001_091714.bin", "last mod"=timestamp(3493796315 s since 1904-01-01), "file name str"="D:\\Data\\Ultrasound\\LSCO\\LSCO22__130814c\\5_Cooling_2nd_try\\September_2014\\091714\\63.82200K_500_2500_2.10000V_0.00000T_Sep17-2014__06-58-35_001_091714.bin", "mod time(min)"=58229938.583333336, "file format"=enum."binary", "power(V)"=2.1, "Magn Field(T) "=0.0}, {"temperature"=63.767, "temperature str"="63.76700", "file path"=path "D:/Data/Ultrasound/LSCO/LSCO22__130814c/5_Cooling_2nd_try/September_2014/091714/63.76700K_500_2500_2.10000V_0.00000T_Sep17-2014__06-59-55_001_091714.bin", "last mod"=timestamp(3493796395 s since 1904-01-01), "file name str"="D:\\Data\\Ultrasound\\LSCO\\LSCO22__130814c\\5_Cooling_2nd_try\\September_2014\\091714\\63.76700K_500_2500_2.10000V_0.00000T_Sep17-2014__06-59-55_001_091714.bin", "mod time(min)"=58229939.916666664, "file format"=enum."binary", "power(V)"=2.1, "Magn Field(T) "=0.0}, {"temperature"=63.708, "temperature str"="63.70800", "file path"=path "D:/Data/Ultrasound/LSCO/LSCO22__130814c/5_Cooling_2nd_try/September_2014/091714/63.70800K_500_2500_2.10000V_0.00000T_Sep17-2014__07-01-14_001_091714.bin", "last mod"=timestamp(3493796474 s since 1904-01-01), "file name str"="D:\\Data\\Ultrasound\\LSCO\\LSCO22__130814c\\5_Cooling_2nd_try\\September_2014\\091714\\63.70800K_500_2500_2.10000V_0.00000T_Sep17-2014__07-01-14_001_091714.bin", "mod time(min)"=58229941.233333334, "file format"=enum."binary", "power(V)"=2.1, "Magn Field(T) "=0.0}, {"temperature"=63.646, "temperature str"="63.64600", "file path"=path "D:/Data/Ultrasound/LSCO/LSCO22__130814c/5_Cooling_2nd_try/September_2014/091714/63.64600K_500_2500_2.10000V_0.00000T_Sep17-2014__07-02-33_001_091714.bin", "last mod"=timestamp(3493796553 s since 1904-01-01), "file name str"="D:\\Data\\Ultrasound\\LSCO\\LSCO22__130814c\\5_Cooling_2nd_try\\September_2014\\091714\\63.64600K_500_2500_2.10000V_0.00000T_Sep17-2014__07-02-33_001_091714.bin", "mod time(min)"=58229942.55, "file format"=enum."binary", "power(V)"=2.1, "Magn Field(T) "=0.0}, {"temperature"=63.59, "temperature str"="63.59000", "file path"=path "D:/Data/Ultrasound/LSCO/LSCO22__130814c/5_Cooling_2nd_try/September_2014/091714/63.59000K_500_2500_2.10000V_0.00000T_Sep17-2014__07-03-53_001_091714.bin", "last mod"=timestamp(3493796633 s since 1904-01-01), "file name str"="D:\\Data\\Ultrasound\\LSCO\\LSCO22__130814c\\5_Cooling_2nd_try\\September_2014\\091714\\63.59000K_500_2500_2.10000V_0.00000T_Sep17-2014__07-03-53_001_091714.bin", "mod time(min)"=58229943.88333333, "file format"=enum."binary", "power(V)"=2.1, "Magn Field(T) "=0.0}, {"temperature"=63.532, "temperature str"="63.53200", "file path"=path "D:/Data/Ultrasound/LSCO/LSCO22__130814c/5_Cooling_2nd_try/September_2014/091714/63.53200K_500_2500_2.10000V_0.00000T_Sep17-2014__07-05-12_001_091714.bin", "last mod"=timestamp(3493796712 s since 1904-01-01), "file name str"="D:\\Data\\Ultrasound\\LSCO\\LSCO22__130814c\\5_Cooling_2nd_try\\September_2014\\091714\\63.53200K_500_2500_2.10000V_0.00000T_Sep17-2014__07-05-12_001_091714.bin", "mod time(min)"=58229945.2, "file format"=enum."binary", "power(V)"=2.1, "Magn Field(T) "=0.0}, {"temperature"=63.472, "temperature str"="63.47200", "file path"=path "D:/Data/Ultrasound/LSCO/LSCO22__130814c/5_Cooling_2nd_try/September_2014/091714/63.47200K_500_2500_2.10000V_0.00000T_Sep17-2014__07-06-31_001_091714.bin", "last mod"=timestamp(3493796791 s since 1904-01-01), "file name str"="D:\\Data\\Ultrasound\\LSCO\\LSCO22__130814c\\5_Cooling_2nd_try\\September_2014\\091714\\63.47200K_500_2500_2.10000V_0.00000T_Sep17-2014__07-06-31_001_091714.bin", "mod time(min)"=58229946.516666666, "file format"=enum."binary", "power(V)"=2.1, "Magn Field(T) "=0.0}, {"temperature"=63.413, "temperature str"="63.41300", "file path"=path "D:/Data/Ultrasound/LSCO/LSCO22__130814c/5_Cooling_2nd_try/September_2014/091714/63.41300K_500_2500_2.10000V_0.00000T_Sep17-2014__07-07-51_001_091714.bin", "last mod"=timestamp(3493796871 s since 1904-01-01), "file name str"="D:\\Data\\Ultrasound\\LSCO\\LSCO22__130814c\\5_Cooling_2nd_try\\September_2014\\091714\\63.41300K_500_2500_2.10000V_0.00000T_Sep17-2014__07-07-51_001_091714.bin", "mod time(min)"=58229947.85, "file format"=enum."binary", "power(V)"=2.1, "Magn Field(T) "=0.0}, {"temperature"=63.355, "temperature str"="63.35500", "file path"=path "D:/Data/Ultrasound/LSCO/LSCO22__130814c/5_Cooling_2nd_try/September_2014/091714/63.35500K_500_2500_2.10000V_0.00000T_Sep17-2014__07-09-10_001_091714.bin", "last mod"=timestamp(3493796950 
